vi "Stop.vi"(8 "error in":errorcluster, 11 "camera.nit in":refnum<class "camera.lvclass">) -> (0 "error out":errorcluster)   [LabVIEW 2020, in "camera.lvclass"]
uses:
  camera.lvclass
  camera.lvclass/camera.ctl
  lib/O-PL.dll
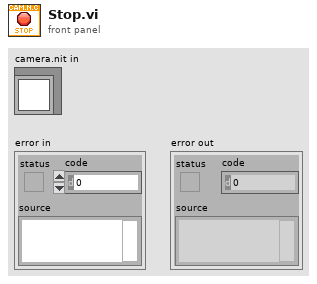
[diagram p1: front panel]
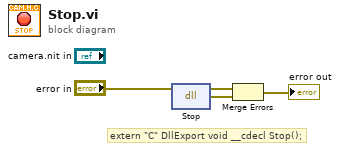
[diagram p0: block diagram]
diagram:
  # "extern \"C\" DllExport void __cdecl Stop();"
  n1 = dll-call lib="C:/Users/pittsburger.SOLARIS/Desktop/v0.8/lib/O-PL.dll" fn="Stop"() -> (error out=w3:errorcluster)  [unwired: 4 in, 1 out]
  n2 = Merge Errors("error in", w3) -> (→"error out":errorcluster)
